vi "Combine data.vi"(1 "name path":path=path "F:/fh/传输D/2015谷粒实验/提取数据/后期处理数据/1-8综合", 2 "base path":path=path "F:/fh/传输D/2015谷粒实验/提取数据/后期处理数据/1-8综合") -> ()   [LabVIEW 2015]
uses:
  <vilib>/Utility/file.llb/Read Delimited Spreadsheet (string).vi
  <vilib>/Utility/file.llb/Write Delimited Spreadsheet (string).vi
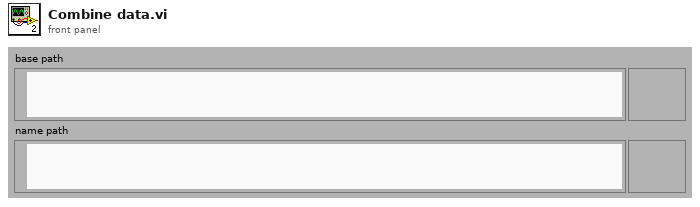
[diagram p1: front panel]
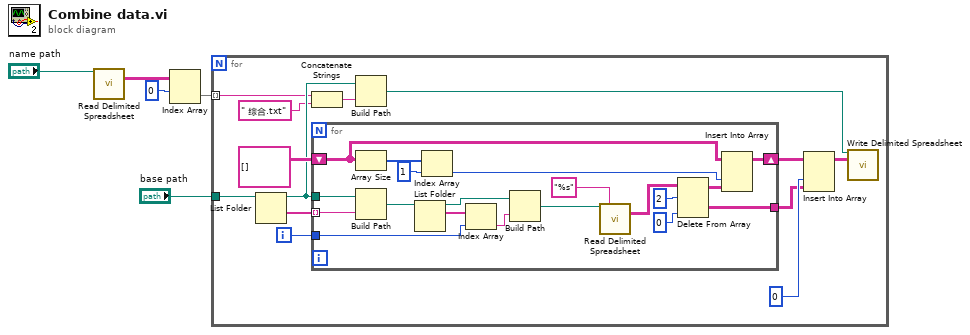
[diagram p0: block diagram]
diagram:
  n1 = call-poly <vilib>:"Read Delimited Spreadsheet.vi"("file path (dialog if empty)"="name path") -> ("all rows"=w3:string[][])  [unwired: 9 in, 5 out]
  n2 = Index Array(array=w3, index (row)=0) -> (element=w1:string[])  [unwired: 1 in]
  n3 = for {
    tunnel: w1 -> [w10] mode=indexing
    tunnel: "base path" -> [w18]
    i -> [w16]
    n4 = List Folder(path=w18) -> (path out=w11:path, folder names=w17:string[])  [unwired: 1 in, 4 out]
    n5 = Concatenate Strings(w10, " 综合.txt" ("string")) -> (w8:string)
    n6 = for {
      tunnel: w17 -> [w36] mode=indexing
      tunnel: w11 -> [w37]
      tunnel: w16 -> [w33]
      shift-right: [w21] -> w14
      shift-left: string[][] [] ("all rows") -> [w26]
      tunnel: [w20] -> w12
      n7 = Array Size(array=w26) -> (size(s)=w25:i32[])
      n8 = Build Path(base path=w37, name or relative path=w36) -> (appended path=w35:path)
      n9 = List Folder(path=w35) -> (path out=w32:path, filenames=w34:string[])  [unwired: 1 in, 4 out]
      n10 = Index Array(array=w25, index=1) -> (element=w23:i32)
      n11 = Index Array(array=w34, index=w33) -> (element=w31:string)
      n12 = Build Path(base path=w32, name or relative path=w31) -> (appended path=w30:path)
      n13 = call-poly <vilib>:"Read Delimited Spreadsheet.vi"("file path (dialog if empty)"=w30, "format (%s)"="%s") -> ("all rows"=w19:string[][])  [unwired: 8 in, 5 out]
      n14 = Delete From Array(array=w19, length=2, index (col)=0 ("disabled index (col)")) -> (deleted portion=w20:string[][], array with subset deleted=w22:string[][])  [unwired: 1 in]
      n15 = Insert Into Array(array=w26, index (col)=w23, new element=w22) -> (w21:string[][])  [unwired: 1 in]
    }
    n16 = Build Path(base path=w11, name or relative path=w8) -> (appended path=w7:path)
    n17 = Insert Into Array(array=w14, index (col)=0 ("disabled index (col)"), new element=w12) -> (w6:string[][])  [unwired: 1 in]
    n18 = call-poly <vilib>:"Write Delimited Spreadsheet.vi"("file path (dialog if empty)"=w7, "2D data"=w6) -> ()  [unwired: 12 in, 2 out]
  }
